vi "spreadsheet string.vi"() -> ()   [LabVIEW 2013]
panel:
  out "spreadsheet string":string
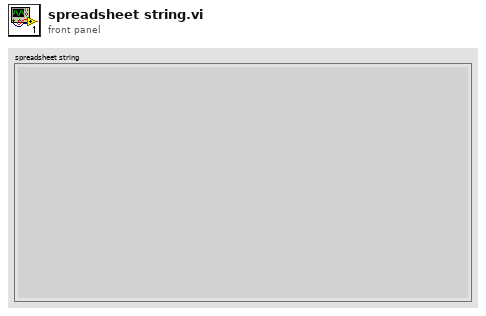
[diagram p1: front panel]
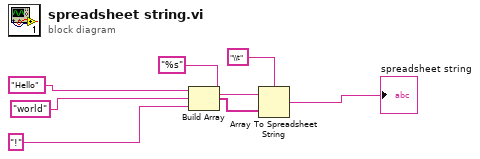
[diagram p0: block diagram]
diagram:
  n1 = Build Array("Hello", "world", "!") -> (w4:string[])
  n2 = Array To Spreadsheet String(delimiter (Tab)="\\t", array=w4, 3:"%s" ("format string")) -> (spreadsheet string=→"spreadsheet string":string)
